vi "ZLIB CRC32__ogtk.vi"(4 "error in (no error)":errorcluster, 6 "buffer":string, 7 "previous crc32":u32) -> (0 "error out":errorcluster, 3 "new crc32":u32)   [LabVIEW 2018]
doc: "Calculates the CRC32 value of a buffer. The previous CRC32 value can be used to pass in the crc32 of a previous buffer in a series of buffers from a data stream."
uses:
  <userlib>/_OpenG.lib/lvzip/lvzlib.dll
panel:
  # "Please visit http://www.OpenG.org to learn about the\nOpen Source LabVIEW software movement.\n\nNOTICE -- YOU MUST LEAVE THIS NOTICE IN PLACE.  PER THE TERMS OF THE LICENSE BELOW, YOU MAY SUBLICENSE THIS SOFTWARE \nIN ANY WAY THAT DOES NOT CONFLICT WITH THIS LICENSE.\n\n### BSD License (http://www.opensource.org/licenses/bsd-license.php) Begin ###\n \nCopyright (C) 2004 Rolf Kalbermatter rolf.kalbermatter@citeng.com\n\nAll rights reserved.\n\nRedistribution and use in source and binary forms, with or without modification, are permitted provided that the following conditions are met:\n\n    * Redistributions of source code must retain the above copyright notice, this list of conditions and the following disclaimer.\n    * Redistributions in binary form must reproduce the above copyright notice, this list of conditions and the following disclaimer in the \n       documentation and/or other materials provided with the distribution.\n    * Neither the name of SciWare, James Kring, Inc., nor the names of its contributors may be used to endorse or promote products derived \n       from this software without specific prior written permission.\n\nTHIS SOFTWARE IS PROVIDED BY THE COPYRIGHT HOLDERS AND CONTRIBUTORS \"AS IS\" AND ANY EXPRESS OR IMPLIED WARRANTIES, \nINCLUDING, BUT NOT LIMITED TO, THE IMPLIED WARRANTIES OF MERCHANTABILITY AND FITNESS FOR A PARTICULAR PURPOSE ARE \nDISCLAIMED. IN NO EVENT SHALL THE COPYRIGHT OWNER OR CONTRIBUTORS BE LIABLE FOR ANY DIRECT, INDIRECT, INCIDENTAL,\n SPECIAL, EXEMPLARY, OR CONSEQUENTIAL DAMAGES (INCLUDING, BUT NOT LIMITED TO, PROCUREMENT OF SUBSTITUTE GOODS OR \nSERVICES; LOSS OF USE, DATA, OR PROFITS; OR BUSINESS INTERRUPTION) HOWEVER CAUSED AND ON ANY THEORY OF LIABILITY, \nWHETHER IN CONTRACT, STRICT LIABILITY, OR TORT (INCLUDING NEGLIGENCE OR OTHERWISE) ARISING IN ANY WAY OUT OF THE USE \nOF THIS SOFTWARE, EVEN IF ADVISED OF THE POSSIBILITY OF SUCH DAMAGE.\n\n### BSD License End ###"
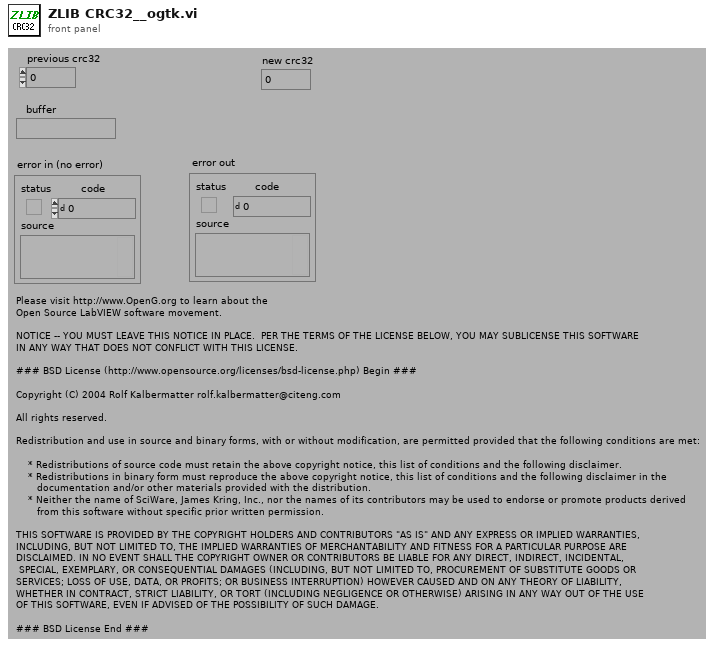
[diagram p1: front panel]
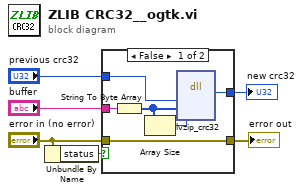
[diagram p0: block diagram]
diagram:
  n1 = Unbundle By Name("error in (no error)") -> ("status"=w6:bool)
  n2 = case shown="False" w6 {
    tunnel: "error in (no error)" -> [w9 w14]
    tunnel: [w9 w14] -> w4
    tunnel: "buffer" -> [w12 _]
    tunnel: [w8 w13] -> w3
    tunnel: "previous crc32" -> [w10 w13]
    frame False {
      n3 = String To Byte Array(string=w12) -> (unsigned byte array=w7:u8[])
      n4 = Array Size(array=w7) -> (size(s)=w11:i32)
      n5 = dll-call lib="C:/Work/OpenG/opengtoolkit/lvzip/source/lvzlib.*" fn="lvzip_crc32"("crc"=w10, "buf"=w7, "len"=w11) -> (w8:u32)  [unwired: 6 in, 2 out]
    }
    frame True {
    }
  }
  "error out" <- w4
  "new crc32" <- w3
